vi "Main.vi"() -> ()   [LabVIEW 2016]
uses:
  XControls/Reference/VI Reference.xctl
  XControls/Class Reference/Class Reference.xctl
panel:
  out "NaN/Path/Refnum? 2":bool
  out "Class Reference 2":refnum<vi>(xcontrol)
  out "NaN/Path/Refnum?":bool
  out "VI Reference 2":refnum<vi>(xcontrol)
  in  "Class Reference":refnum<vi>(xcontrol)
  in  "VI Reference":refnum<vi>(xcontrol)
  in  "Execute Script":bool
  in  "stop":bool
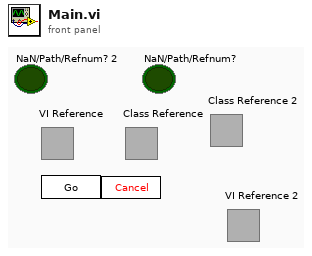
[diagram p1: front panel]
types:
  T1 = enum8{"Enabled", "Disabled", "Disabled and Grayed Out"}
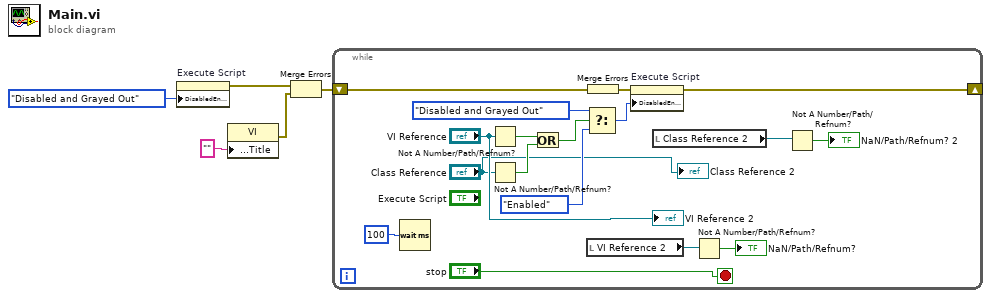
[diagram p0: block diagram]
diagram:
  n1 = property on="Execute Script" class="Bool"("DisabledEnum"=T1."Disabled and Grayed Out" ("Disabled")) -> (error out=w4:errorcluster)  [unwired: 2 in, 1 out]
  n2 = property class="VI"("Front Panel.Title"="" ("Front Panel Window:Title")) -> (error out=w1:errorcluster)  [unwired: 2 in, 1 out]
  n3 = Merge Errors(w4, w1) -> (w3:errorcluster)
  n4 = while {
    shift-right: [w21] -> _
    shift-left: w3 -> [w20]
    stop <- "stop" stop-if-true
    n5 = Wait (ms)(milliseconds to wait=u32 100) -> ()  [unwired: 1 out]
    n6 = Not A Number/Path/Refnum?(number/path/refnum="VI Reference") -> (NaN/Path/Refnum?=w14:bool)
    n7 = Not A Number/Path/Refnum?(number/path/refnum="Class Reference") -> (NaN/Path/Refnum?=w12:bool)
    n8 = Or(x=w14, y=w12) -> (x .or. y?=w13:bool)
    n9 = Select(t=T1."Disabled and Grayed Out" ("f"), s=w13, f=T1."Enabled" ("Disabled")) -> (s? t:f=w22:T1)
    n10 = local read "VI Reference 2"() -> (w10:refnum<vi>)
    n11 = Merge Errors(w20) -> (w19:errorcluster)
    n12 = property on="Execute Script" class="Bool"(error in=w19, "DisabledEnum"=w22) -> (error out=w21:errorcluster)  [unwired: 1 in, 1 out]
    n13 = local read "Class Reference 2"() -> (w6:refnum<vi>)
    n14 = Not A Number/Path/Refnum?(number/path/refnum=w10) -> (NaN/Path/Refnum?=→"NaN/Path/Refnum?":bool)
    n15 = Not A Number/Path/Refnum?(number/path/refnum=w6) -> (NaN/Path/Refnum?=→"NaN/Path/Refnum? 2":bool)
    "VI Reference 2" <- "VI Reference"
    "Class Reference 2" <- "Class Reference"
  }
